vi "SQL_添加主键为ID其余为字符字段的表.vi"(8 "error IO":errorcluster, 9 "connection reference":T1, 10 "字段名(字符字段)":string[](array[string]), 11 "表名":string="test") -> (0 "error out":errorcluster caption="错误输出", 2 "字段名(字符字段) 输出":string[](array[string]), 3 "SQL_在指定表中添加列":string)   [LabVIEW 2014]
doc: "该模板用于创建子VI。"
uses:
  <vilib>/addons/database/Connection.llb/Conn ObjectReference.ctl
  <vilib>/addons/database/Connection.llb/Conn Execute.vi
  <vilib>/addons/database/Recordset.llb/Rec Destroy - Connection.vi
  <vilib>/addons/database/NI_Database_API.lvlib
  <vilib>/addons/database/Connection.llb/DB Tools Open Connec (String).vi
panel:
  # "varchar括号中的数值最大255"
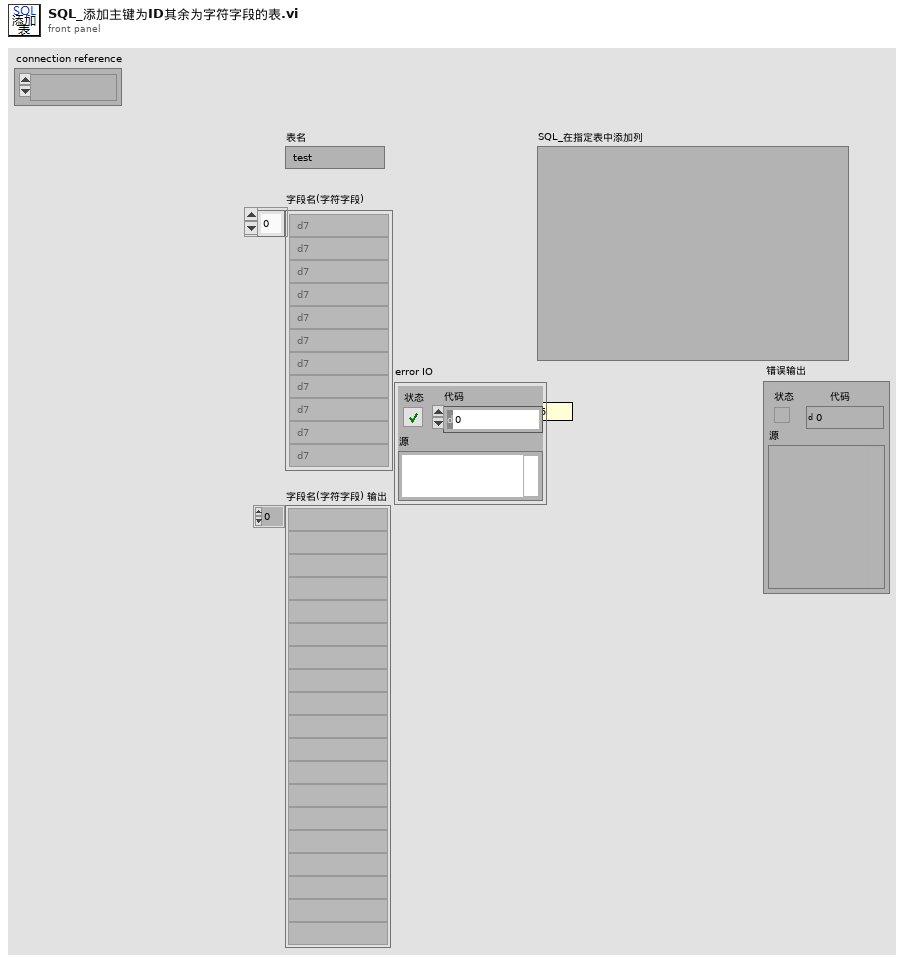
[diagram p1: front panel]
types:
  T1 = typedef "NI_Database_API.lvlib/Conn ObjectReference.ctl" = refnum<k1>
  T2 = typedef "NI_Database_API.lvlib/Rec ObjectReference.ctl" = refnum<k1>
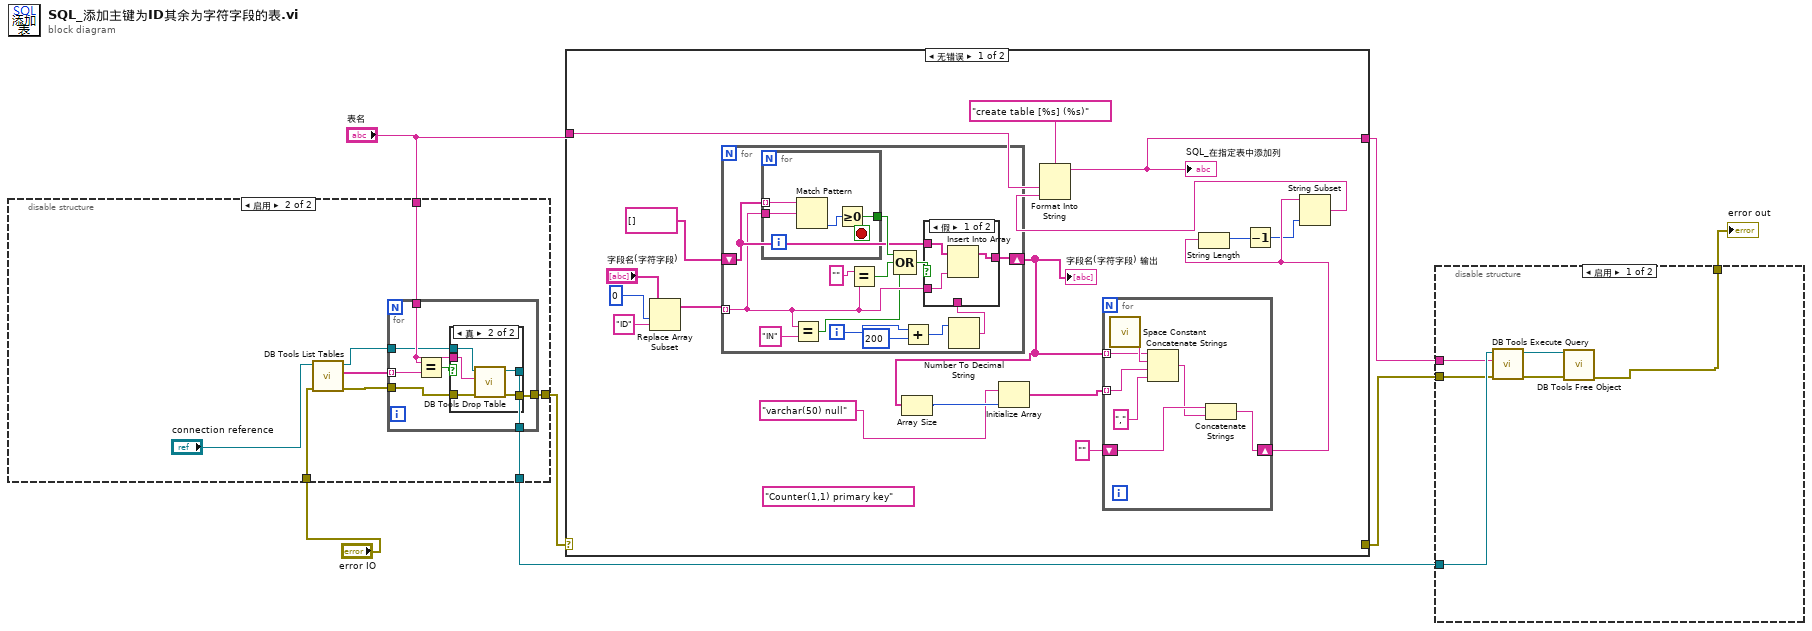
[diagram p0: block diagram]
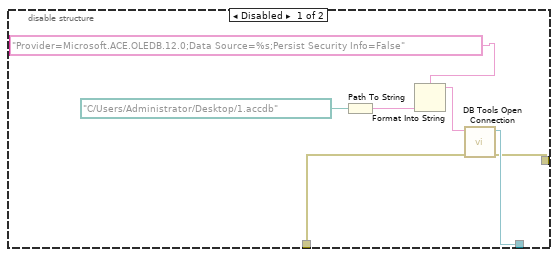
[diagram p3: hidden frame]
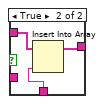
[diagram p5: hidden frame]
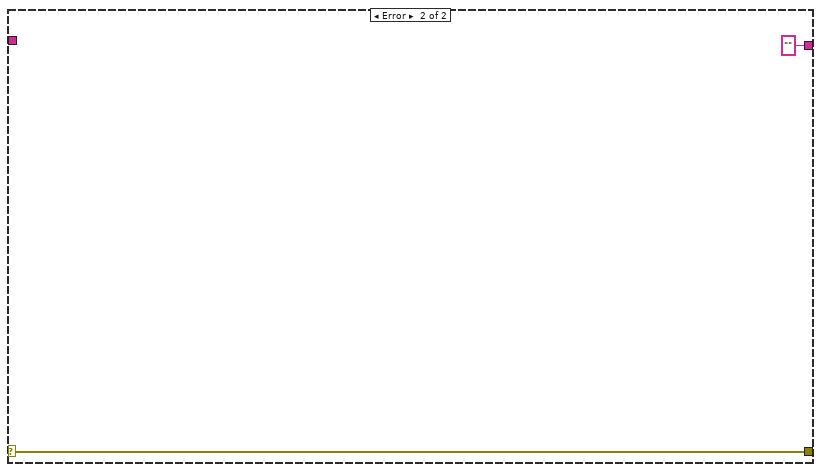
[diagram p6: hidden frame]
diagram:
  n1 = disable-structure shown="启用" {
    disable-tunnel: [w11 w16] -> w6
    disable-tunnel: "表名" -> [_ w21]
    disable-tunnel: "error IO" -> [w9 w17]
    disable-tunnel: [w8 w15] -> w1
    frame Disabled {
      n2 = Path To String(path=path "C:/Users/Administrator/Desktop/1.accdb" ("路径")) -> (string=w14:string)
      n3 = Format Into String(format string="Provider=Microsoft.ACE.OLEDB.12.0;Data Source=%s;Persist Security Info=False" ("初始字符串"), w14) -> (resulting string=w13:string)  [unwired: 2 in, 1 out]
      n4 = call-poly <vilib>:"DB Tools Open Connection.vi"("error in (no error)"=w9, "connection information"=w13) -> ("error out"=w8:errorcluster, "connection reference"=w11:T1)  [unwired: 6 in]
    }
    frame Enabled {
      n5 = call <vilib>:"DB Tools List Tables.vi"("error in (no error)"=w17, "connection reference"="connection reference") -> ("error out"=w18:errorcluster, "tables"=w20:string[], "connection reference out"=w19:T1)  [unwired: 3 in]
      n6 = for {
        tunnel: w21 -> [w27]
        tunnel: w20 -> [w29] mode=indexing
        tunnel: w19 -> [w26]
        tunnel: w18 -> [w25]
        tunnel: [w24] -> w16
        tunnel: [w23] -> w15
        n7 = Equal?(x=w27, y=w29) -> (x = y?=w28:bool)
        n8 = case shown="真" w28 {
          tunnel: w27 -> [_ w36]
          tunnel: w26 -> [w31 w35]
          tunnel: w25 -> [w30 w34]
          tunnel: [w31 w33] -> w24
          tunnel: [w30 w32] -> w23
          frame False {
          }
          frame True {
            n9 = call <vilib>:"DB Tools Drop Table.vi"("error in (no error)"=w34, "table"=w36, "connection reference"=w35) -> ("error out"=w32:errorcluster, "connection reference out"=w33:T1)  [unwired: 5 in]
          }
        }
      }
    }
  }
  n10 = case shown="无错误" w1 {
    selector: w1 -> [_ w85]
    tunnel: [_ w85] -> w5
    tunnel: [w44 ""] -> w7
    tunnel: "表名" -> [w43 _]
    frame No Error {
      (unwired) "Counter(1,1) primary key"
      n11 = Replace Array Subset(array="字段名(字符字段)", new element="ID", index=0 ("索引")) -> (w39:string[])
      n12 = for {
        tunnel: w39 -> [w56] mode=indexing
        shift-right: [w57] -> w37
        shift-left: string[] [] -> [w58]
        i -> [w65]
        n13 = for {
          tunnel: w56 -> [w70]
          tunnel: w58 -> [w69] mode=indexing
          tunnel: [w67] -> w60
          stop <- w67 stop-if-true
          n14 = Match Pattern(string=w69, regular expression=w70) -> (offset past match=w68:i32)  [unwired: 1 in, 3 out]
          n15 = Greater Or Equal To 0?(x=w68) -> (x >= 0?=w67:bool)
        }
        n16 = Equal?(x=w56, y="IN") -> (x = y?=w54:bool)
        n17 = Equal?(x="", y=w56) -> (x = y?=w59:bool)
        n18 = Compound Arithmetic op=OR(w60, w59, w54) -> (w61:bool)
        n19 = Add(x=w65, y=200) -> (x+y=w63:i32)
        n20 = Number To Decimal String(number=w63) -> (decimal integer string=w62:string)  [unwired: 1 in]
        n21 = case shown="假" w61 {
          tunnel: w56 -> [w71 _]
          tunnel: [w72 w75] -> w57
          tunnel: w58 -> [w73 w76]
          tunnel: w62 -> [_ w74]
          frame False {
            n22 = Insert Into Array(array=w73, new element=w71) -> (w72:string[])  [unwired: 1 in]
          }
          frame True {
            n23 = Insert Into Array(array=w76, new element=w74) -> (w75:string[])  [unwired: 1 in]
          }
        }
      }
      "字段名(字符字段) 输出" <- w37
      n24 = Array Size(array=w37) -> (size(s)=w47:i32)
      n25 = Initialize Array("varchar(50) null", w47) -> (w45:string[])
      n26 = for {
        tunnel: w45 -> [w83] mode=indexing
        shift-right: [w79] -> w50
        shift-left: "" -> [w81]
        tunnel: w37 -> [w77] mode=indexing
        n27 = call <vilib>:"Space Constant.vi"() -> ("String"=w78:string)
        n28 = Concatenate Strings(w77, w78, w83, ",") -> (w80:string)
        n29 = Concatenate Strings(w81, w80) -> (w79:string)
      }
      n30 = String Length(string=w50) -> (length=w51:i32)
      n31 = Decrement(x=w51) -> (x-1=w48:i32)
      n32 = String Subset(string=w50, length (rest)=w48) -> (substring=w49:string)  [unwired: 1 in]
      n33 = Format Into String(format string="create table [%s] (%s)", w43, w49) -> (resulting string=w44:string)  [unwired: 2 in, 1 out]
      "SQL_在指定表中添加列" <- w44
    }
    frame Error {
    }
  }
  n34 = disable-structure shown="启用" {
    disable-tunnel: w6 -> [w90 _]
    disable-tunnel: w7 -> [w88 _]
    disable-tunnel: w5 -> [w87 _]
    disable-tunnel: [w86 _] -> w4
    frame Enabled {
      n35 = call-poly <vilib>:"DB Tools Execute Query.vi"("error in (no error)"=w87, "SQL query"=w88, "connection reference"=w90) -> ("error out"=w89:errorcluster, "recordset reference"=w91:T2)  [unwired: 5 in]
      n36 = call-poly <vilib>:"DB Tools Free Object.vi"("error in (no error)"=w89, "recordset reference"=w91) -> ("error out"=w86:errorcluster)  [unwired: 8 in, 1 out]
    }
    frame Disabled {
    }
  }
  "error out" <- w4
